vi "Reg to BCD.vi"(1 "Input Registers":u16[](array[numeric])) -> (0 "BCD Value":ext)   [LabVIEW 2019, in "Userlib.lvlib"]
uses:
  Userlib.lvlib
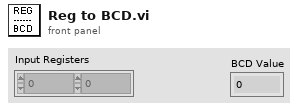
[diagram p1: front panel]
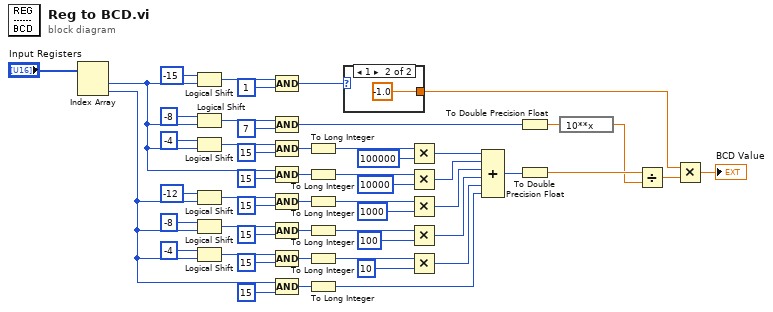
[diagram p0: block diagram]
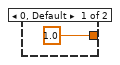
[diagram p2: hidden frame]
diagram:
  n1 = Index Array(array="Input Registers") -> (element #1=w2:u16, element #2=w4:u16)  [unwired: 2 in]
  n2 = Logical Shift(y=i16 -15, x=w2) -> (x << y=w8:u16)
  n3 = Logical Shift(y=i16 -8, x=w2) -> (x << y=w7:u16)
  n4 = Logical Shift(y=i16 -4, x=w2) -> (x << y=w13:u16)
  n5 = Logical Shift(y=i16 -12, x=w4) -> (x << y=w6:u16)
  n6 = Logical Shift(y=i16 -8, x=w4) -> (x << y=w5:u16)
  n7 = Logical Shift(y=i16 -4, x=w4) -> (x << y=w15:u16)
  n8 = Compound Arithmetic op=AND(w8, u16 1 ("mask (16)")) -> (w23:u16)
  n9 = Compound Arithmetic op=AND(w7, u16 7 ("mask (16)")) -> (w34:u16)
  n10 = Compound Arithmetic op=AND(w13, u16 15 ("mask (16)")) -> (w29:u16)
  n11 = Compound Arithmetic op=AND(w2, u16 15 ("mask (16)")) -> (w28:u16)
  n12 = Compound Arithmetic op=AND(w6, u16 15 ("value")) -> (w27:u16)
  n13 = Compound Arithmetic op=AND(w5, u16 15 ("value")) -> (w26:u16)
  n14 = Compound Arithmetic op=AND(w15, u16 15 ("value")) -> (w25:u16)
  n15 = Compound Arithmetic op=AND(w4, u16 15 ("value")) -> (w24:u16)
  n16 = To Long Integer(number=w29) -> (32bit integer=w49:i32)
  n17 = To Long Integer(number=w28) -> (32bit integer=w48:i32)
  n18 = To Long Integer(number=w27) -> (32bit integer=w41:i32)
  n19 = To Long Integer(number=w26) -> (32bit integer=w40:i32)
  n20 = To Long Integer(number=w25) -> (32bit integer=w38:i32)
  n21 = To Long Integer(number=w24) -> (32bit integer=w39:i32)
  n22 = case shown="1" w23 {
    tunnel: [1.0 -1.0] -> w21
    frame 0, Default {
    }
    frame 1 {
    }
  }
  n23 = Multiply(x=w49, y=100000) -> (x*y=w47:i32)
  n24 = Multiply(x=w48, y=10000) -> (x*y=w46:i32)
  n25 = Multiply(x=w41, y=1000) -> (x*y=w37:i32)
  n26 = Multiply(x=w40, y=100) -> (x*y=w36:i32)
  n27 = Multiply(x=w38, y=10) -> (x*y=w35:i32)
  n28 = Compound Arithmetic op=ADD(w47, w46, w37, w36, w35, w39) -> (w45:i32)
  n29 = To Double Precision Float(number=w34) -> (double precision float=w44:dbl)
  n30 = To Double Precision Float(number=w45) -> (double precision float=w43:dbl)
  n31 = expression code="10**x"(w44) -> (w42:dbl)
  n32 = Divide(x=w43, y=w42) -> (x/y=w22:dbl)
  n33 = Multiply(x=w21, y=w22) -> (x*y=→"BCD Value":dbl)
